vi "Tx.vi"(8 "error in (no error)":errorcluster, 11 "Framework in":refnum<class "Framework.lvclass">) -> (0 "error out":errorcluster, 3 "Framework out":refnum<class "Framework.lvclass">)   [LabVIEW 2017, in "DSF Core.lvlib" / "Framework.lvclass"]
uses:
  Framework.lvclass
  Framework.lvclass/Framework.ctl
  Scheduler/Scheduler.lvclass
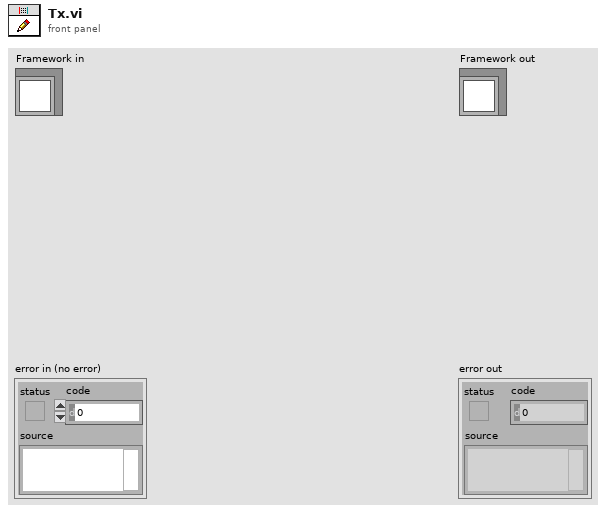
[diagram p1: front panel]
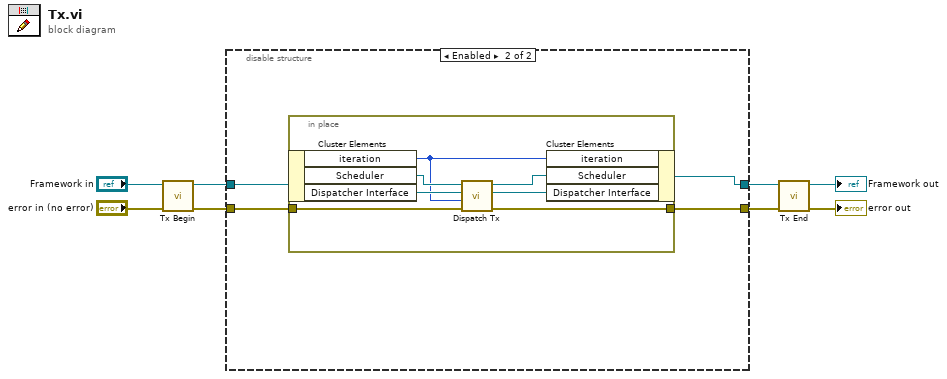
[diagram p0: block diagram]
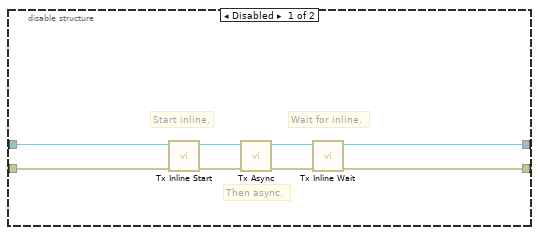
[diagram p2: hidden frame]
diagram:
  n1 = call "Tx Begin.vi"("error in (no error)"="error in (no error)", "Framework in"="Framework in") -> ("error out"=w5:errorcluster, "Framework out"=w6:refnum<class "Framework.lvclass">)  [unwired: 8 in]
  n2 = disable-structure shown="Enabled" {
    disable-tunnel: w6 -> [w12 w20]
    disable-tunnel: w5 -> [w11 w19]
    disable-tunnel: [w10 w17] -> w4
    disable-tunnel: [w9 w18] -> w3
    frame Disabled {
      # "Wait for inline."
      # "Start inline."
      # "Then async."
      n3 = call "Tx Inline Start.vi"("error in (no error)"=w11, "Framework in"=w12) -> ("error out"=w14:errorcluster, "Framework out"=w13:refnum<class "Framework.lvclass">)  [unwired: 8 in]
      n4 = call "Tx Async.vi"("error in (no error)"=w14, "Framework in"=w13) -> ("error out"=w16:errorcluster, "Framework out"=w15:refnum<class "Framework.lvclass">)  [unwired: 8 in]
      n5 = call "Tx Inline Wait.vi"("error in (no error)"=w16, "Framework in"=w15) -> ("error out"=w9:errorcluster, "Framework out"=w10:refnum<class "Framework.lvclass">)  [unwired: 8 in]
    }
    frame Enabled {
      n6 = in-place {
        in-place-border: w19 -> [w26]
        in-place-border: [w25] -> w18
        n7 = in-place-cluster #1(w20) -> ("iteration"=w21:u64, "Scheduler"=w27:refnum<class "Scheduler.lvclass">, "Dispatcher Interface"=w23:refnum<class "Dispatcher Interface.lvclass">)
        n8 = call "Dispatch Tx.vi"("error in (no error)"=w26, "framework iteration"=w21, "Dispatcher Interface in"=w23, "Scheduler in"=w27) -> ("error out"=w25:errorcluster, "Dispatcher Interface out"=w22:refnum<class "Dispatcher Interface.lvclass">, "Scheduler out"=w24:refnum<class "Scheduler.lvclass">)  [unwired: 5 in]
        n9 = in-place-cluster #1("iteration"=w21, "Scheduler"=w24, "Dispatcher Interface"=w22) -> (w17:refnum<class "Framework.lvclass">)
      }
    }
  }
  n10 = call "Tx End.vi"("error in (no error)"=w3, "Framework in"=w4) -> ("error out"=→"error out":errorcluster, "Framework out"=→"Framework out":refnum<class "Framework.lvclass">)  [unwired: 8 in]
